vi "view.vi"() -> ()   [LabVIEW 2018]
uses:
  control/clusterCustomString.ctl
  <vilib>/Utility/miscctls.llb/LVPointTypeDef.ctl
  control/enumFgvFunction.ctl
  control/enumTcpCommand.ctl
  <vilib>/Utility/sysdir.llb/System Directory Type.ctl
  control/clusterPeriod.ctl
panel:
  out "Get Whisper(Recv ms)":u32(graph)
  in  "File Name":string
  in  "Save":bool
  out "connect?":bool
  out "rx(ms)":u32
  out "tx(ms)":u32
  out "retry":i32
  in  "Tab Control":enum32{"monitor1", "monitor2", "RecipeLab"}(tab)
  out "value 1-1":T1[](array[typedef]) {"value" format="%#_6f"}
  out "chart 1-1":dbl[][](graph)
  in  "display 1-1":cluster{"subject":u16}[](array[cluster]) {"subject" items=["current_0", "current_1", "current_2", "current_3", "refSpeed_0", "refSpeed_1", "refSpeed_2", "refSpeed_3", "in_rpm_0", "in_rpm_1", "in_rpm_2", "in_rpm_3", "out_rpm_0", "out_rpm_1", "out_rpm_2", "out_rpm_3", "temperature_0", "temperature_1", "temperature_2", "temperature_3", "position_0", "position_1", "position_2", "position_3", "", "", "", "", "", ""]}
  out "chart 1-2":dbl[][](graph)
  out "value 1-2":T1[](array[typedef]) {"value" format="%#_6f"}
  in  "display 1-2":cluster{"subject":u16}[](array[cluster]) {"subject" items=["current_0", "current_1", "current_2", "current_3", "refSpeed_0", "refSpeed_1", "refSpeed_2", "refSpeed_3", "in_rpm_0", "in_rpm_1", "in_rpm_2", "in_rpm_3", "out_rpm_0", "out_rpm_1", "out_rpm_2", "out_rpm_3", "temperature_0", "temperature_1", "temperature_2", "temperature_3", "position_0", "position_1", "position_2", "position_3", "", "", "", "", "", ""]}
  out "chart 2-1":dbl[][](graph)
  out "value 2-1":T1[](array[typedef]) {"value" format="%#_6f"}
  in  "display 2-1":cluster{"subject":u16}[](array[cluster])
  out "chart 2-2":dbl[][](graph)
  out "value 2-2":T1[](array[typedef]) {"value" format="%#_6f"}
  in  "display 2-2":cluster{"subject":u16}[](array[cluster])
  out "stop":bool
  out "rx_packet ts":timestamp format="%<%H:%M:%S%3u>T"
  out "tx_packet ts":timestamp format="%<%H:%M:%S%3u>T"
  in  "send":bool
  in  "tcp rx close?":bool
  in  "port":u16=10300
  in  "address":string="127.0.0.1"
  out "rx_packet":string
  out "tx_packet":string
  in  "saving?":bool
  in  "tx string":string
  out "Whisper":T1[](array[typedef]) {"value" format="%#_6f"}
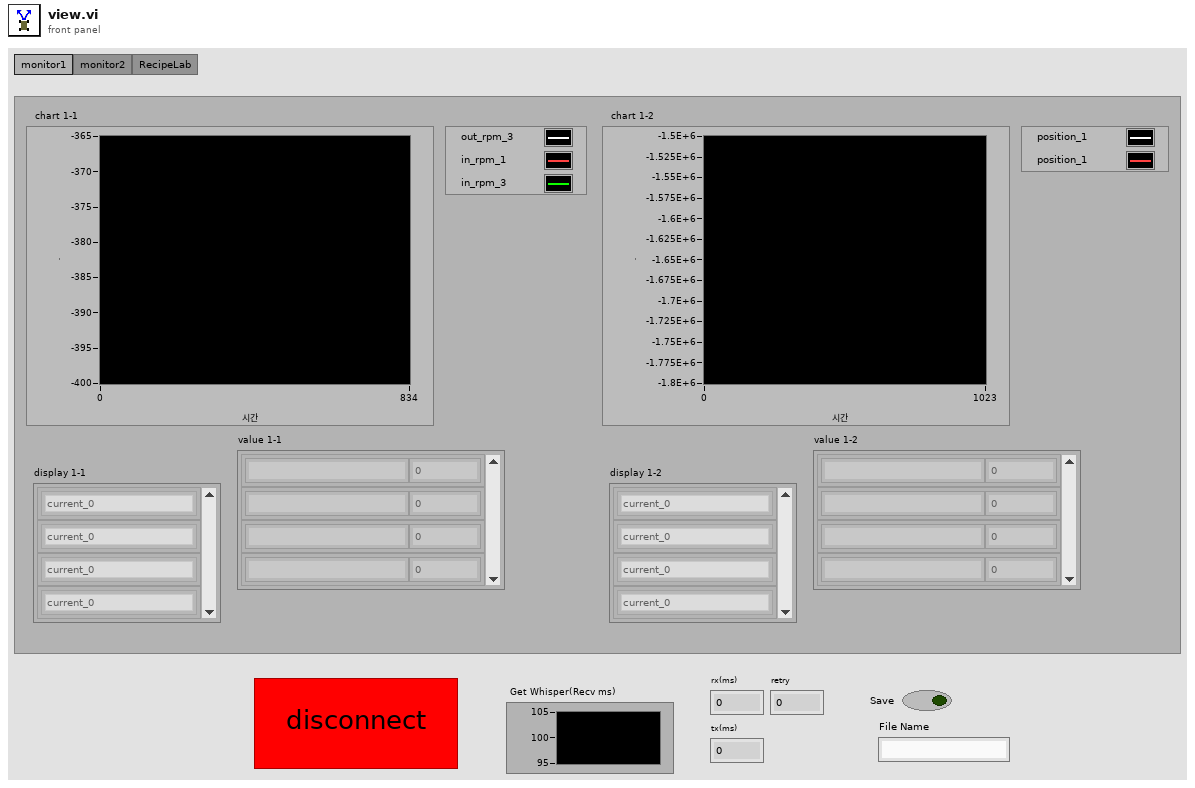
[diagram p1: front panel]
types:
  T1 = typedef "clusterCustomString.ctl" = cluster{"subject":string, "value":dbl}
  T2 = enum32{"invalid app kind", "Development System", "Run Time System", "Student Edition", "Embedded LabVIEW", "Evaluation", "Custom"}
  T3 = typedef "LVPointTypeDef.ctl" = cluster{"Horizontal":i16, "Vertical":i16}
  T4 = typedef "enumFgvFunction.ctl" = enum16{"Open", "Read", "Check", "Write", "Close"}
  T5 = cluster{"subject":u64, "subject":i64, "val_dbl":dbl}[]
  T6 = typedef "System Directory Type.ctl" = i32
  T7 = typedef "clusterPeriod.ctl" = cluster{"Period(ms)":i32}
  T8 = typedef "enumTcpCommand.ctl" = enum16{"None", "Stop", "E-Stop", "Set Position Control Mode", "Set Jog Control Mode", "Set Control Mode", "Set Jog Control Profile Parameter", "Set Position Control Profile Parameter", "Set Jog State", "Set Position", "Start Position Control", "Get Total State", "Get Platform State", "Get Sensor State", "Get Position State", "Init Platform", "Get Whisper State", "Set Sensor"}
  T9 = enum16{"Standard", "Buffered", "CRLF", "Immediate"}
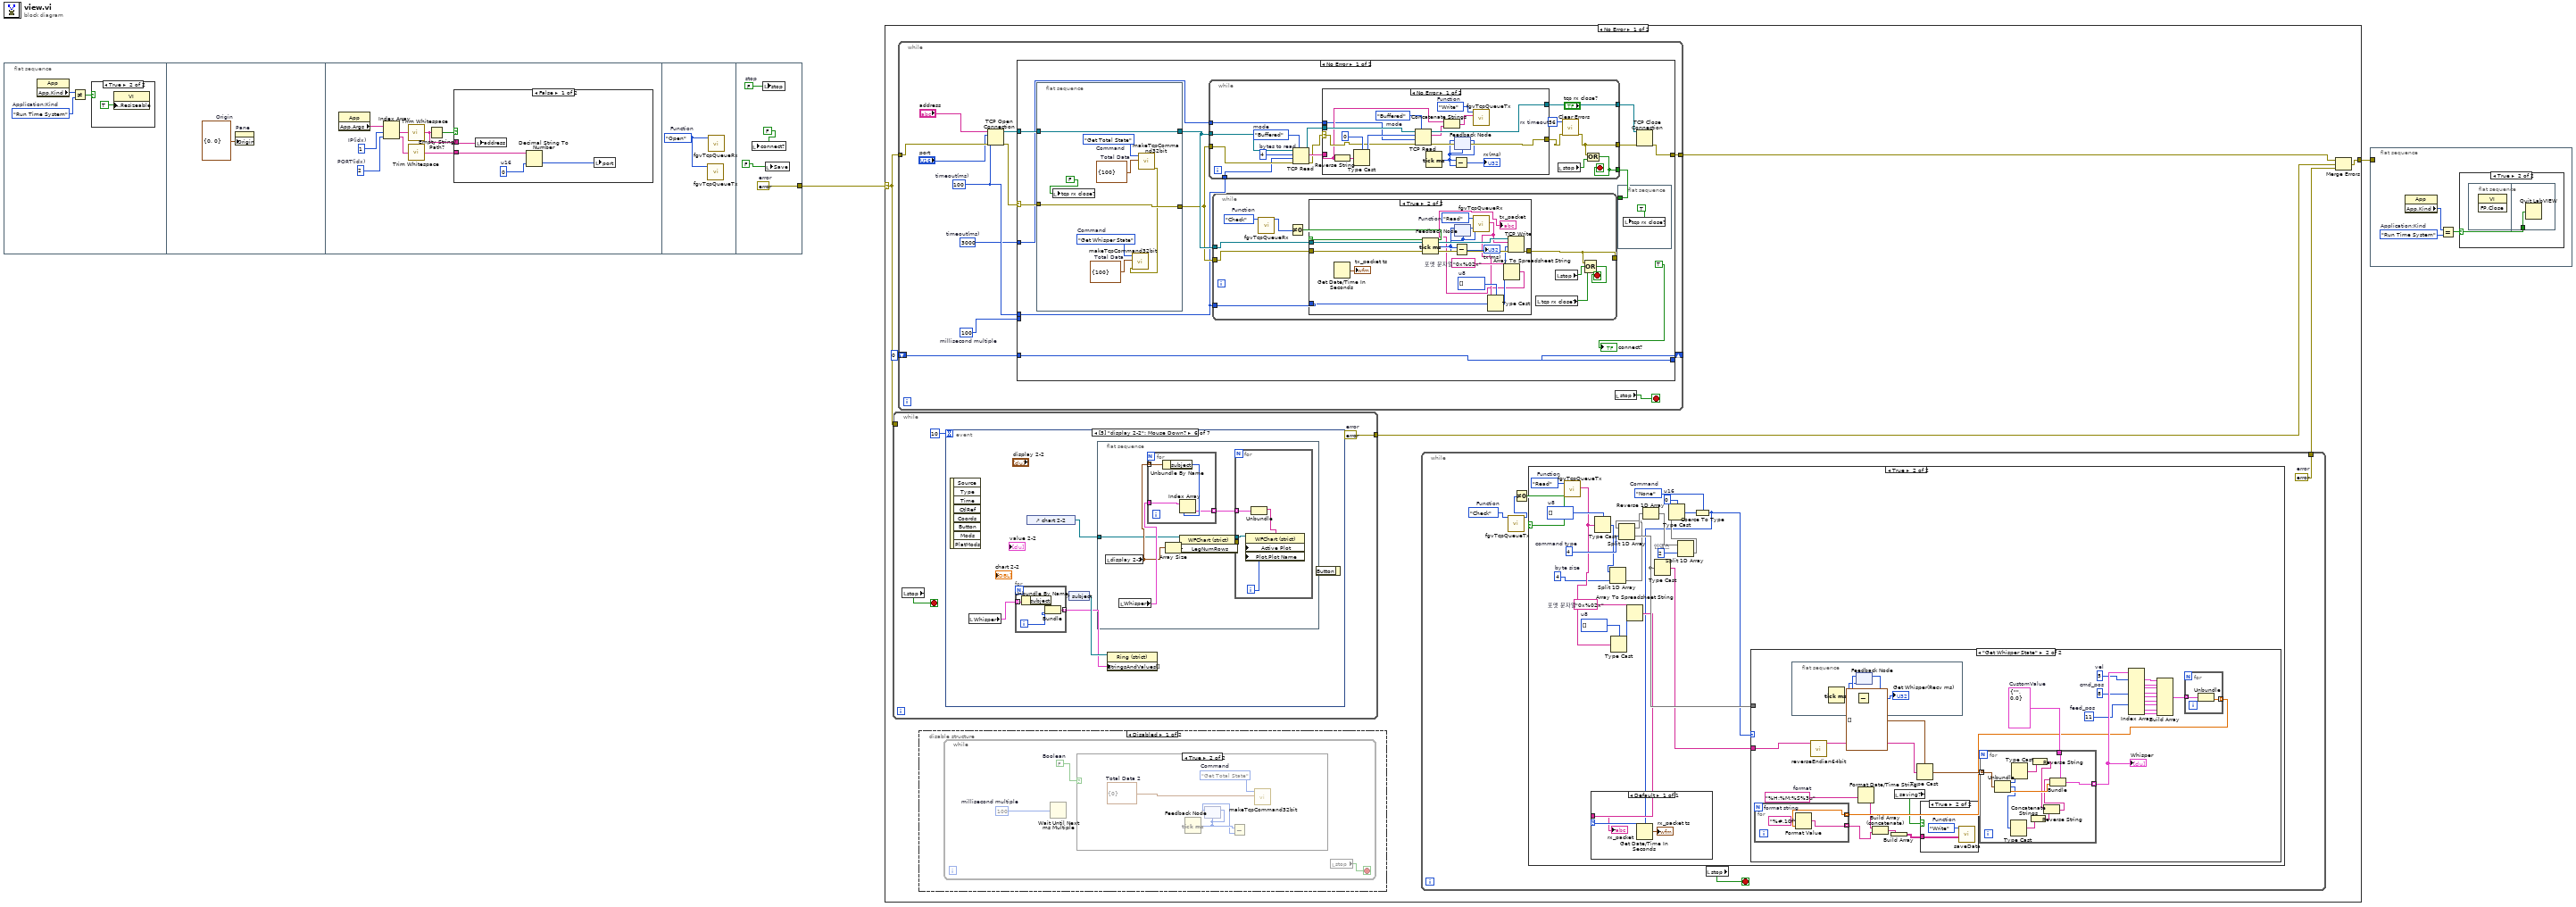
[diagram p0: block diagram]
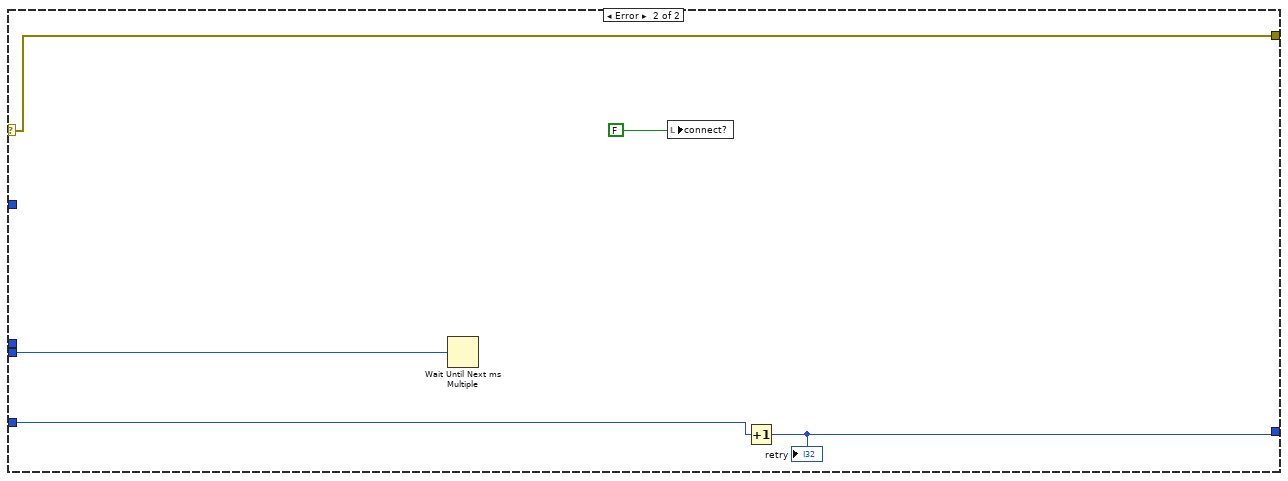
[diagram p9: hidden frame]
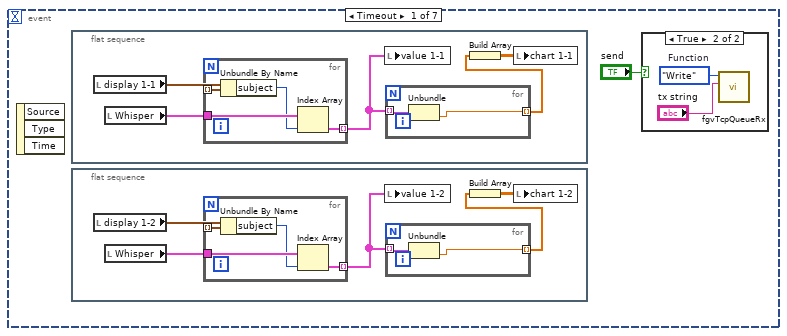
[diagram p10: hidden frame]
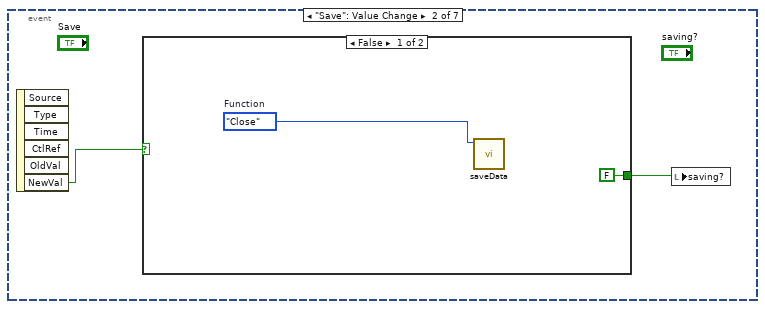
[diagram p12: hidden frame]
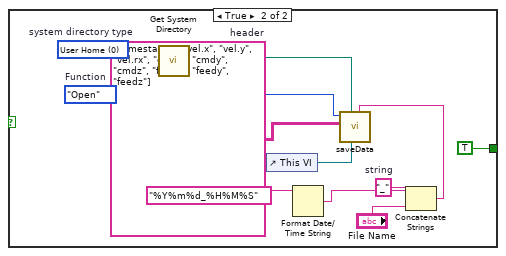
[diagram p13: hidden frame]
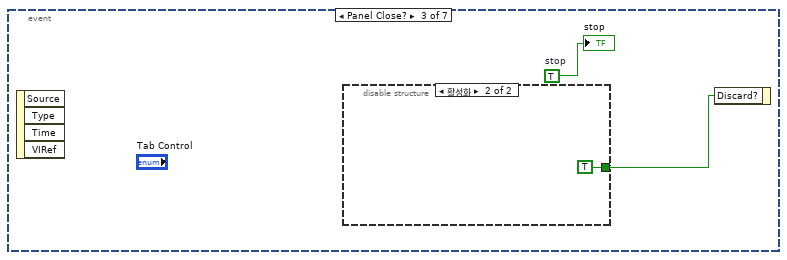
[diagram p14: hidden frame]
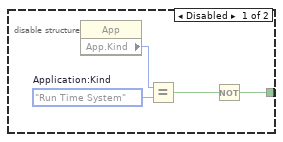
[diagram p15: hidden frame]
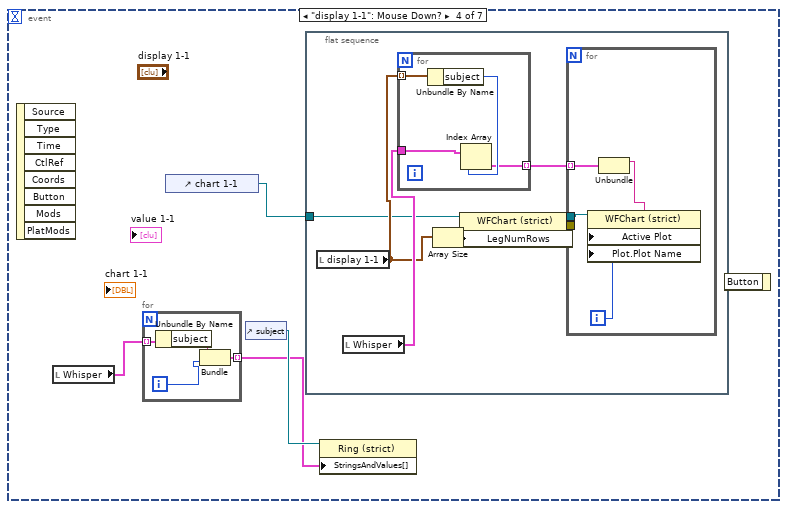
[diagram p16: hidden frame]
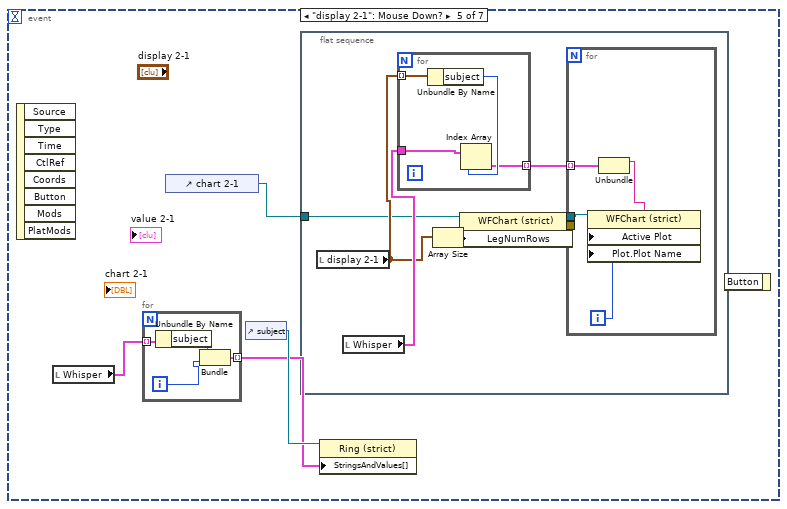
[diagram p17: hidden frame]
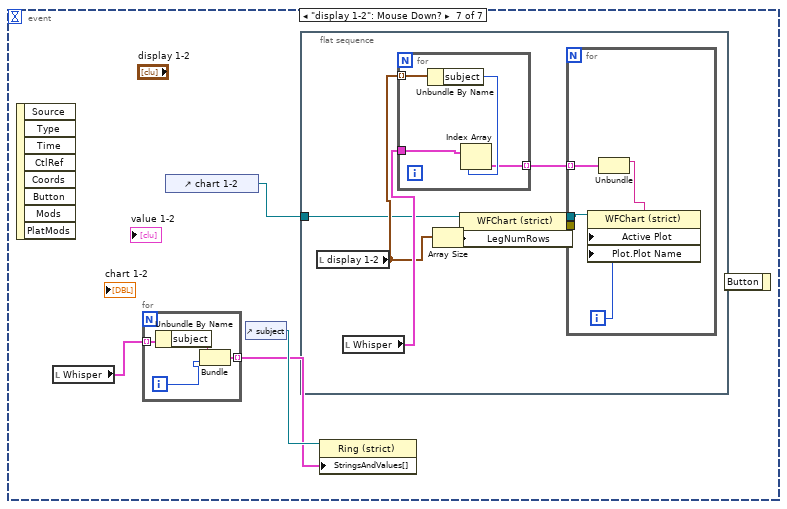
[diagram p18: hidden frame]
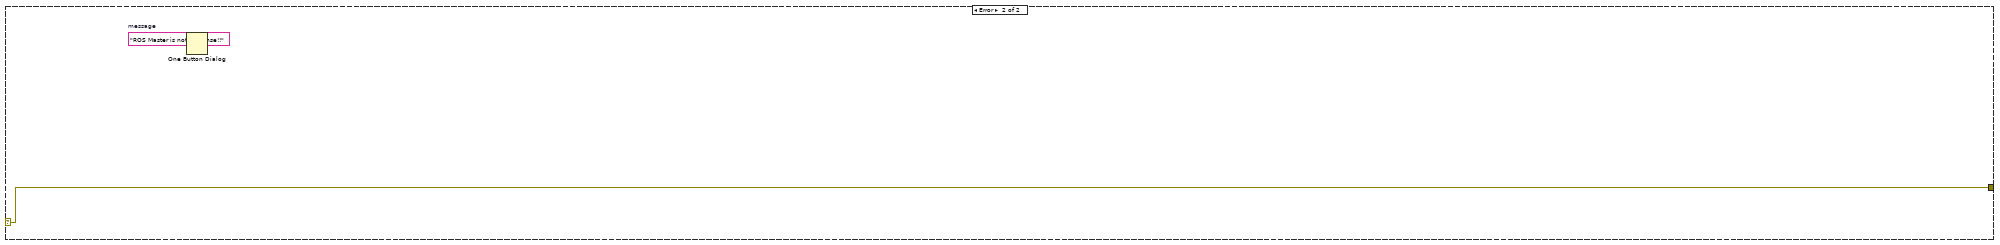
[diagram p19: hidden frame]
diagram:
  n1 = flat-sequence {
    tunnel: [w23] -> w1
    frame #0 {
      w3 = T2."Run Time System"  # Application:Kind
      n2 = property class="App"() -> ("App.Kind"=w4:T2)  [unwired: 2 in, 2 out]
      n3 = Not Equal?(x=w4, y=w3) -> (x != y?=w5:bool)
      n4 = case shown="True" w5 {
        frame False {
        }
        frame True {
          n5 = property class="VI"("Front Panel.Resizeable"=TRUE) -> ()  [unwired: 2 in, 2 out]
        }
      }
    }
    frame #1 {
      w7 = T3 {"Horizontal"=0, "Vertical"=0}  # Origin
      n6 = property on="Pane" class="Pane"("Origin"=w7) -> ()  [unwired: 2 in, 2 out]
    }
    frame #2 {
      w13 = 2  # PORT(idx)
      w14 = 1  # IP(idx)
      n7 = property class="App"() -> ("App.Args"=w15:string[])  [unwired: 2 in, 2 out]
      n8 = Index Array(array=w15, index #1=w14, index #2=w13) -> (element #1=w12:string, element #2=w11:string)
      n9 = call <vilib>:"Trim Whitespace.vi"("string"=w12) -> ("trimmed string"=w10:string)  [unwired: 1 in]
      n10 = call <vilib>:"Trim Whitespace.vi"("string"=w11) -> ("trimmed string"=w9:string)  [unwired: 1 in]
      n11 = Empty String/Path?(string/path=w10) -> (empty?=w8:bool)
      n12 = case shown="False" w8 {
        tunnel: w10 -> [w19 _]
        tunnel: w9 -> [w18 _]
        frame False {
          w16 = u16 0  # u16
          n13 = local write "address"(w19) -> ()
          n14 = Decimal String To Number(string=w18, default (0L)=w16) -> (number=w17:u16)  [unwired: 1 in, 1 out]
          n15 = local write "port"(w17) -> ()
        }
        frame True {
        }
      }
    }
    frame #3 {
      w20 = enumFgvFunction."Open"  # Function
      n16 = call "fgvTcpQueueTx.vi"("Function"=w20) -> ()  [unwired: 8 in, 3 out]
      n17 = call "fgvTcpQueueRx.vi"("Function"=w20) -> ()  [unwired: 8 in, 3 out]
    }
    frame #4 {
      w23 = errorcluster {"status"=FALSE, "code"=0, "source"=""}  # error
      w24 = FALSE  # stop
      n18 = local write "connect?"(FALSE) -> ()
      n19 = local write "stop"(w24) -> ()
      n20 = local write "Save"(FALSE) -> ()
    }
  }
  n21 = case shown="No Error" w1 {
    selector: w1 -> [w28 w348]
    tunnel: [w29 w348] -> w2
    frame No Error {
      n22 = while {
        tunnel: w28 -> [_]
        tunnel: [w209] -> w30
        stop <- w211 stop-if-true
        w209 = errorcluster {"status"=FALSE, "code"=0, "source"=""}  # error
        n23 = local read "stop"() -> (w211:bool)
        n24 = event shown="[5] \"display 2-2\": Mouse Down?" {
          selector: _ -> [_ _ _ _ _ _ _]
          dyn-events: _ -> [_ _ _ _ _ _ _]
          timeout: 10 -> [_ _ _ _ _ _ _]
          event Timeout {
            n25 = event-data() -> ()  [unwired: 1 in, 3 out]
            n26 = flat-sequence {
              frame #0 {
                n27 = local read "display 1-1"() -> (w228:cluster{"subject":u16}[])
                n28 = local read "Whisper"() -> (w227:T1[])
                n29 = for {
                  tunnel: w228 -> [w233] mode=indexing
                  tunnel: w227 -> [w234]
                  tunnel: [w231] -> w225 mode=indexing
                  n30 = Unbundle By Name(w233) -> ("subject"=w232:u16)
                  n31 = Index Array(array=w234, index=w232) -> (element=w231:T1)
                }
                n32 = local write "value 1-1"(w225) -> ()
                n33 = for {
                  tunnel: w225 -> [w230] mode=indexing
                  tunnel: [w229] -> w226 mode=indexing
                  n34 = Unbundle(w230) -> ("value"=w229:dbl)  [unwired: 1 out]
                }
                n35 = Build Array(w226) -> (w224:dbl[][])
                n36 = local write "chart 1-1"(w224) -> ()
              }
            }
            n37 = flat-sequence {
              frame #0 {
                n38 = local read "display 1-2"() -> (w217:cluster{"subject":u16}[])
                n39 = local read "Whisper"() -> (w216:T1[])
                n40 = for {
                  tunnel: w217 -> [w222] mode=indexing
                  tunnel: w216 -> [w223]
                  tunnel: [w220] -> w214 mode=indexing
                  n41 = Unbundle By Name(w222) -> ("subject"=w221:u16)
                  n42 = Index Array(array=w223, index=w221) -> (element=w220:T1)
                }
                n43 = local write "value 1-2"(w214) -> ()
                n44 = for {
                  tunnel: w214 -> [w219] mode=indexing
                  tunnel: [w218] -> w215 mode=indexing
                  n45 = Unbundle(w219) -> ("value"=w218:dbl)  [unwired: 1 out]
                }
                n46 = Build Array(w215) -> (w213:dbl[][])
                n47 = local write "chart 1-2"(w213) -> ()
              }
            }
            n48 = case shown="True" "send" {
              frame False {
              }
              frame True {
                w236 = enumFgvFunction."Write"  # Function
                n49 = call "fgvTcpQueueRx.vi"("Write"="tx string", "Function"=w236) -> ()  [unwired: 7 in, 3 out]
              }
            }
          }
          event "Save": Value Change {
            n50 = event-data() -> ("NewVal"=w238:bool)  [unwired: 1 in, 5 out]
            n51 = case shown="False" w238 {
              tunnel: [FALSE TRUE] -> w237
              frame False {
                w240 = enumFgvFunction."Close"  # Function
                n52 = call "saveData.vi"("Function"=w240) -> ()  [unwired: 8 in, 3 out]
              }
              frame True {
                w241 = "_"  # string
                w246 = string[][] [["timestamp", "vel.x", "vel.y", "vel.rx", "cmdx", "cmdy", "cmdz", "feedx", "feedy", "feedz"]]  # header
                w249 = T6 0 items=["User Home"=0, "User Desktop"=1, "User Documents"=2, "User Application Data"=3, "User Preferences"=4, "User Temporary"=5, "Public Documents"=6, "Public Application Data"=7, "Public Preferences"=8, "Public Cache"=13, "System Core Libraries"=9, "System Installed Libraries"=10, "Application Files"=11, "Boot Volume Root"=12]  # system directory type
                w251 = enumFgvFunction."Open"  # Function
                n53 = call <vilib>:"Get System Directory.vi"("system directory type"=w249) -> ("system directory"=w248:path)  [unwired: 10 in]
                n54 = control-ref of="This VI"() -> (w245:refnum<vi>)
                n55 = Format Date/Time String(time format string (%c)="%Y%m%d_%H%M%S") -> (date/time string=w244:string)  [unwired: 2 in]
                n56 = Concatenate Strings(w244, w241, "File Name") -> (w242:string)
                n57 = call "saveData.vi"("file name"=w242, "이미지 저장 VI"=w245, "file path 경로"=w248, "header"=w246, "Function"=w251) -> ()  [unwired: 4 in, 3 out]
              }
            }
            n58 = local write "saving?"(w237) -> ()
          }
          event Panel Close? {
            w252 = TRUE  # stop
            n59 = event-data() -> ()  [unwired: 1 in, 4 out]
            n60 = disable-structure shown="활성화" {
              disable-tunnel: [w254 TRUE] -> w253
              frame Disabled {
                w256 = T2."Run Time System"  # Application:Kind
                n61 = property class="App"() -> ("App.Kind"=w257:T2)  [unwired: 2 in, 2 out]
                n62 = Equal?(x=w257, y=w256) -> (x = y?=w255:bool)
                n63 = Not(x=w255) -> (.not. x?=w254:bool)
              }
              frame Enabled {
              }
            }
            n64 = event-data("Discard?"=w253) -> ()  [unwired: 1 in, 1 out]
            "stop" <- w252
          }
          event "display 1-1": Mouse Down? {
            n65 = event-data() -> ()  [unwired: 1 in, 8 out]
            n66 = local read "Whisper"() -> (w261:T1[])
            n67 = for {
              tunnel: [w278] -> w260 mode=indexing
              tunnel: w261 -> [w277] mode=indexing
              i -> [w279]
              n68 = Unbundle By Name(w277) -> ("subject"=w280:string)
              n69 = Bundle("subject"=w280, w279) -> (w278:cluster{"subject":string, i32})  [unwired: 1 in]
            }
            n70 = control-ref of="chart 1-1"() -> (w259:refnum<vi>)
            n71 = control-ref of="subject"() -> (w262:refnum<vi>)
            n72 = flat-sequence {
              tunnel: w259 -> [w263]
              frame #0 {
                n73 = local read "display 1-1"() -> (w265:cluster{"subject":u16}[])
                n74 = local read "Whisper"() -> (w266:T1[])
                n75 = for {
                  tunnel: w265 -> [w271] mode=indexing
                  tunnel: w266 -> [w272]
                  tunnel: [w269] -> w264 mode=indexing
                  n76 = Unbundle By Name(w271) -> ("subject"=w270:u16)
                  n77 = Index Array(array=w272, index=w270) -> (element=w269:T1)
                }
                n78 = Array Size(array=w265) -> (size(s)=w268:i32)
                n79 = property on="프로퍼티 노드" class="WFChart (strict)"(reference=w263, "LegNumRows"=w268) -> (error out=w267:errorcluster)  [unwired: 1 in, 1 out]
                n80 = for {
                  tunnel: w267 -> [_]
                  tunnel: w264 -> [w275] mode=indexing
                  tunnel: w263 -> [w273]
                  i -> [w276]
                  n81 = Unbundle(w275) -> ("subject"=w274:string)  [unwired: 1 out]
                  n82 = property on="프로퍼티 노드" class="WFChart (strict)"(reference=w273, "Active Plot"=w276, "Plot.Plot Name"=w274) -> ()  [unwired: 1 in, 2 out]
                }
              }
            }
            n83 = property class="Ring (strict)"(reference=w262, "StringsAndValues[]"=w260) -> ()  [unwired: 1 in, 2 out]
            n84 = event-data() -> ()  [unwired: 2 in, 1 out]
          }
          event "display 2-1": Mouse Down? {
            n85 = event-data() -> ()  [unwired: 1 in, 8 out]
            n86 = local read "Whisper"() -> (w283:T1[])
            n87 = for {
              tunnel: [w300] -> w282 mode=indexing
              tunnel: w283 -> [w299] mode=indexing
              i -> [w301]
              n88 = Unbundle By Name(w299) -> ("subject"=w302:string)
              n89 = Bundle("subject"=w302, w301) -> (w300:cluster{"subject":string, i32})  [unwired: 1 in]
            }
            n90 = control-ref of="chart 2-1"() -> (w281:refnum<vi>)
            n91 = control-ref of="subject"() -> (w284:refnum<vi>)
            n92 = flat-sequence {
              tunnel: w281 -> [w285]
              frame #0 {
                n93 = local read "display 2-1"() -> (w287:cluster{"subject":u16}[])
                n94 = local read "Whisper"() -> (w288:T1[])
                n95 = for {
                  tunnel: w287 -> [w293] mode=indexing
                  tunnel: w288 -> [w294]
                  tunnel: [w291] -> w286 mode=indexing
                  n96 = Unbundle By Name(w293) -> ("subject"=w292:u16)
                  n97 = Index Array(array=w294, index=w292) -> (element=w291:T1)
                }
                n98 = Array Size(array=w287) -> (size(s)=w290:i32)
                n99 = property on="프로퍼티 노드" class="WFChart (strict)"(reference=w285, "LegNumRows"=w290) -> (error out=w289:errorcluster)  [unwired: 1 in, 1 out]
                n100 = for {
                  tunnel: w289 -> [_]
                  tunnel: w286 -> [w297] mode=indexing
                  tunnel: w285 -> [w295]
                  i -> [w298]
                  n101 = Unbundle(w297) -> ("subject"=w296:string)  [unwired: 1 out]
                  n102 = property on="프로퍼티 노드" class="WFChart (strict)"(reference=w295, "Active Plot"=w298, "Plot.Plot Name"=w296) -> ()  [unwired: 1 in, 2 out]
                }
              }
            }
            n103 = property class="Ring (strict)"(reference=w284, "StringsAndValues[]"=w282) -> ()  [unwired: 1 in, 2 out]
            n104 = event-data() -> ()  [unwired: 2 in, 1 out]
          }
          event "display 2-2": Mouse Down? {
            n105 = event-data() -> ()  [unwired: 1 in, 8 out]
            n106 = local read "Whisper"() -> (w305:T1[])
            n107 = for {
              tunnel: [w322] -> w304 mode=indexing
              tunnel: w305 -> [w321] mode=indexing
              i -> [w323]
              n108 = Unbundle By Name(w321) -> ("subject"=w324:string)
              n109 = Bundle("subject"=w324, w323) -> (w322:cluster{"subject":string, i32})  [unwired: 1 in]
            }
            n110 = control-ref of="chart 2-2"() -> (w303:refnum<vi>)
            n111 = control-ref of="subject"() -> (w306:refnum<vi>)
            n112 = flat-sequence {
              tunnel: w303 -> [w307]
              frame #0 {
                n113 = local read "display 2-2"() -> (w309:cluster{"subject":u16}[])
                n114 = local read "Whisper"() -> (w310:T1[])
                n115 = for {
                  tunnel: w309 -> [w315] mode=indexing
                  tunnel: w310 -> [w316]
                  tunnel: [w313] -> w308 mode=indexing
                  n116 = Unbundle By Name(w315) -> ("subject"=w314:u16)
                  n117 = Index Array(array=w316, index=w314) -> (element=w313:T1)
                }
                n118 = Array Size(array=w309) -> (size(s)=w312:i32)
                n119 = property on="프로퍼티 노드" class="WFChart (strict)"(reference=w307, "LegNumRows"=w312) -> (error out=w311:errorcluster)  [unwired: 1 in, 1 out]
                n120 = for {
                  tunnel: w311 -> [_]
                  tunnel: w308 -> [w319] mode=indexing
                  tunnel: w307 -> [w317]
                  i -> [w320]
                  n121 = Unbundle(w319) -> ("subject"=w318:string)  [unwired: 1 out]
                  n122 = property on="프로퍼티 노드" class="WFChart (strict)"(reference=w317, "Active Plot"=w320, "Plot.Plot Name"=w318) -> ()  [unwired: 1 in, 2 out]
                }
              }
            }
            n123 = property class="Ring (strict)"(reference=w306, "StringsAndValues[]"=w304) -> ()  [unwired: 1 in, 2 out]
            n124 = event-data() -> ()  [unwired: 2 in, 1 out]
          }
          event "display 1-2": Mouse Down? {
            n125 = event-data() -> ()  [unwired: 1 in, 8 out]
            n126 = local read "Whisper"() -> (w327:T1[])
            n127 = for {
              tunnel: [w344] -> w326 mode=indexing
              tunnel: w327 -> [w343] mode=indexing
              i -> [w345]
              n128 = Unbundle By Name(w343) -> ("subject"=w346:string)
              n129 = Bundle("subject"=w346, w345) -> (w344:cluster{"subject":string, i32})  [unwired: 1 in]
            }
            n130 = control-ref of="chart 1-2"() -> (w325:refnum<vi>)
            n131 = control-ref of="subject"() -> (w328:refnum<vi>)
            n132 = flat-sequence {
              tunnel: w325 -> [w329]
              frame #0 {
                n133 = local read "display 1-2"() -> (w331:cluster{"subject":u16}[])
                n134 = local read "Whisper"() -> (w332:T1[])
                n135 = for {
                  tunnel: w331 -> [w337] mode=indexing
                  tunnel: w332 -> [w338]
                  tunnel: [w335] -> w330 mode=indexing
                  n136 = Unbundle By Name(w337) -> ("subject"=w336:u16)
                  n137 = Index Array(array=w338, index=w336) -> (element=w335:T1)
                }
                n138 = Array Size(array=w331) -> (size(s)=w334:i32)
                n139 = property on="프로퍼티 노드" class="WFChart (strict)"(reference=w329, "LegNumRows"=w334) -> (error out=w333:errorcluster)  [unwired: 1 in, 1 out]
                n140 = for {
                  tunnel: w333 -> [_]
                  tunnel: w330 -> [w341] mode=indexing
                  tunnel: w329 -> [w339]
                  i -> [w342]
                  n141 = Unbundle(w341) -> ("subject"=w340:string)  [unwired: 1 out]
                  n142 = property on="프로퍼티 노드" class="WFChart (strict)"(reference=w339, "Active Plot"=w342, "Plot.Plot Name"=w340) -> ()  [unwired: 1 in, 2 out]
                }
              }
            }
            n143 = property class="Ring (strict)"(reference=w328, "StringsAndValues[]"=w326) -> ()  [unwired: 1 in, 2 out]
            n144 = event-data() -> ()  [unwired: 2 in, 1 out]
          }
        }
      }
      n145 = while {
        tunnel: w28 -> [w123]
        tunnel: [w122] -> w27
        shift-right: [w117] -> _
        shift-left: 0 -> [w116]
        stop <- w124 stop-if-true
        w113 = 3000  # timeout(ms)
        w115 = u32 100  # millisecond multiple
        w114 = 100  # timeout(ms)
        n146 = TCP Open Connection(address="address", remote port or service name="port", timeout ms (60000)=w114, error in (no error)=w123) -> (connection ID=w119:refnum<k5>, error out=w118:errorcluster)  [unwired: 1 in]
        n147 = case shown="No Error" w118 {
          selector: w118 -> [w128 w208]
          tunnel: [w135 w208] -> w122
          tunnel: w119 -> [w130 _]
          tunnel: [w133 w206] -> w117
          tunnel: w116 -> [w133 w207]
          tunnel: w115 -> [_ w204]
          tunnel: w114 -> [w127 _]
          tunnel: w113 -> [w126 _]
          frame No Error {
            n148 = flat-sequence {
              tunnel: [w145] -> w131
              tunnel: w130 -> [w145]
              tunnel: [w144] -> w129
              tunnel: w128 -> [w144]
              frame #0 {
                w141 = T7 {"Period(ms)"=100}  # Total Data
                w140 = enumTcpCommand."Get Whisper State"  # Command
                w142 = T7 {"Period(ms)"=100}  # Total Data
                w143 = enumTcpCommand."Get Total State"  # Command
                n149 = local write "tcp rx close?"(FALSE) -> ()
                n150 = call "makeTcpCommand32bit.vi"("Variant"=w142, "Command"=w143) -> ("error out"=w139:errorcluster)  [unwired: 7 in, 2 out]
                n151 = call "makeTcpCommand32bit.vi"("error in"=w139, "Variant"=w141, "Command"=w140) -> ()  [unwired: 6 in, 3 out]
              }
            }
            n152 = while {
              tunnel: w129 -> [w185]
              tunnel: [w175] -> w136
              tunnel: w131 -> [w184]
              tunnel: [w178] -> w134
              tunnel: w127 -> [w173]
              tunnel: w126 -> [w172]
              tunnel: [w171] -> w125
              stop <- w171 stop-if-true
              w174 = 56  # rx timeout
              w182 = 4  # bytes to read
              w183 = T9."Buffered"  # mode
              n153 = TCP Read(connection ID=w184, bytes to read=w182, error in (no error)=w185, 7:w183, 9:w173) -> (connection ID out=w180:refnum<k5>, data out=w179:string, error out=w177:errorcluster)
              n154 = case shown="No Error" w177 {
                selector: w177 -> [w193 w203]
                tunnel: w180 -> [w200 w202]
                tunnel: w179 -> [w189 _]
                tunnel: [w196 w202] -> w178
                tunnel: [w195 w203] -> w176
                tunnel: w172 -> [w186 _]
                frame No Error {
                  w194 = enumFgvFunction."Write"  # Function
                  w201 = T9."Buffered"  # mode
                  n155 = Reverse String(1:w189) -> (0:w199:string)
                  n156 = Type Cast(type=0, x=w199) -> (*(type *) &x=w198:i32)
                  n157 = TCP Read(connection ID=w200, bytes to read=w198, error in (no error)=w193, 7:w201, 9:w186) -> (connection ID out=w196:refnum<k5>, data out=w188:string, error out=w195:errorcluster)
                  n158 = Tick Count (ms)() -> (millisecond timer value=w191:u32)
                  n159 = Concatenate Strings(w189, w188) -> (w187:string)
                  n160 = feedback #1(w191) -> (w190:u32)
                  n161 = Subtract(x=w191, y=w190) -> (x-y=→"rx(ms)":u32)
                  n162 = feedback-in #1(w191) -> ()
                  n163 = call "fgvTcpQueueTx.vi"("Write"=w187, "Function"=w194) -> ()  [unwired: 7 in, 3 out]
                }
                frame Error {
                }
              }
              n164 = local read "stop"() -> (w181:bool)
              n165 = call <vilib>:"Clear Errors.vi"("error in (no error)"=w176, "specific error code to clear (0: all)"=w174) -> ("error out"=w175:errorcluster)  [unwired: 4 in, 1 out]
              n166 = Compound Arithmetic op=OR(w175, w181) -> (w171:bool)
            }
            n167 = while {
              tunnel: w129 -> [w147]
              tunnel: [w155] -> _
              tunnel: w131 -> [w149]
              tunnel: w127 -> [w148]
              stop <- w153 stop-if-true
              w152 = enumFgvFunction."Check"  # Function
              n168 = call "fgvTcpQueueRx.vi"("Function"=w152) -> ("Count"=w151:i32)  [unwired: 8 in, 2 out]
              n169 = Not Equal To 0?(x=w151) -> (x != 0?=w150:bool)
              n170 = case shown="True" w150 {
                tunnel: [w156 w170] -> w155
                tunnel: w147 -> [w156 w169]
                tunnel: w149 -> [_ w168]
                tunnel: w148 -> [_ w158]
                frame False {
                }
                frame True {
                  w163 = "0x%02x"  # 포맷 문자열
                  w161 = u8[] []  # u8
                  w167 = enumFgvFunction."Read"  # Function
                  n171 = Get Date/Time In Seconds() -> (seconds since 1Jan1904=→"tx_packet ts":timestamp)
                  n172 = Tick Count (ms)() -> (millisecond timer value=w165:u32)
                  n173 = feedback #2(w165) -> (w164:u32)
                  n174 = Subtract(x=w165, y=w164) -> (x-y=→"tx(ms)":u32)
                  n175 = feedback-in #2(w165) -> ()
                  n176 = call "fgvTcpQueueRx.vi"("Function"=w167) -> ("Read"=w160:string)  [unwired: 8 in, 2 out]
                  n177 = Type Cast(type=w161, x=w160) -> (*(type *) &x=w162:u8[])
                  n178 = Array To Spreadsheet String(array=w162, 3:w163) -> (spreadsheet string=→"tx_packet":string)  [unwired: 1 in]
                  n179 = TCP Write(connection ID=w168, data in=w160, error in (no error)=w169, 9:w158) -> (error out=w170:errorcluster)  [unwired: 2 out]
                }
              }
              n180 = local read "tcp rx close?"() -> (w146:bool)
              n181 = local read "stop"() -> (w154:bool)
              n182 = Compound Arithmetic op=OR(w155, w154, w146) -> (w153:bool)
            }
            n183 = flat-sequence {
              tunnel: w125 -> [_]
              frame #0 {
                n184 = local write "tcp rx close?"(TRUE) -> ()
              }
            }
            n185 = TCP Close Connection(connection ID=w134, error in (no error)=w136) -> (error out=w135:errorcluster)  [unwired: 1 in, 1 out]
            "connect?" <- TRUE
          }
          frame Error {
            n186 = Wait Until Next ms Multiple(millisecond multiple=w204) -> ()  [unwired: 1 out]
            n187 = local write "connect?"(FALSE) -> ()
            n188 = Increment(x=w207) -> (x+1=w206:i32)
            "retry" <- w206
          }
        }
        n189 = local read "stop"() -> (w124:bool)
      }
      n190 = disable-structure shown="Disabled" {
        frame Disabled {
          n191 = while {
            stop <- w32 stop-if-true
            w31 = FALSE  # Boolean
            w33 = u32 100  # millisecond multiple
            n192 = Wait Until Next ms Multiple(millisecond multiple=w33) -> ()  [unwired: 1 out]
            n193 = case shown="True" w31 {
              frame False {
              }
              frame True {
                w37 = T7 {"Period(ms)"=0}  # Total Data 2
                w36 = enumTcpCommand."Get Total State"  # Command
                n194 = Tick Count (ms)() -> (millisecond timer value=w35:u32)
                n195 = feedback-in #3(w35) -> ()
                n196 = feedback #3(w35) -> (w34:u32)
                n197 = Subtract(x=w35, y=w34) -> ()  [unwired: 1 out]
                n198 = call "makeTcpCommand32bit.vi"("Variant"=w37, "Command"=w36) -> ()  [unwired: 7 in, 3 out]
              }
            }
            n199 = local read "stop"() -> (w32:bool)
          }
        }
        frame Enabled {
        }
      }
      n200 = while {
        tunnel: [w38] -> w25
        stop <- w41 stop-if-true
        w38 = errorcluster {"status"=FALSE, "code"=0, "source"=""}  # error
        w42 = enumFgvFunction."Check"  # Function
        n201 = call "fgvTcpQueueTx.vi"("Function"=w42) -> ("Count"=w40:i32)  [unwired: 8 in, 2 out]
        n202 = Not Equal To 0?(x=w40) -> (x != 0?=w39:bool)
        n203 = case shown="True" w39 {
          frame False {
          }
          frame True {
            w46 = 2  # 인덱스
            w48 = 4  # byte size
            w53 = "0x%02x"  # 포맷 문자열
            w55 = u8[] []  # u8
            w44 = u16 0  # u16
            w59 = enumTcpCommand."None"  # Command
            w61 = 4  # command type
            w62 = u8[] []  # u8
            w63 = enumFgvFunction."Read"  # Function
            n204 = call "fgvTcpQueueTx.vi"("Function"=w63) -> ("Read"=w51:string)  [unwired: 8 in, 2 out]
            n205 = Type Cast(type=w62, x=w51) -> (*(type *) &x=w50:u8[])
            n206 = Split 1D Array(array=w50, index=w48) -> (second subarray=w49:u8[])  [unwired: 1 out]
            n207 = Type Cast(type=w55, x=w51) -> (*(type *) &x=w54:u8[])
            n208 = Split 1D Array(array=w49, index=w61) -> (first subarray=w60:u8[], second subarray=w57:u8[])
            n209 = Array To Spreadsheet String(array=w54, 3:w53) -> (spreadsheet string=w52:string)  [unwired: 1 in]
            n210 = Reverse 1D Array(array=w60) -> (reversed array=w47:u8[])
            n211 = Type Cast(x=w57) -> (*(type *) &x=w56:string)  [unwired: 1 in]
            n212 = Split 1D Array(array=w47, index=w46) -> (second subarray=w45:u8[])  [unwired: 1 out]
            n213 = Type Cast(type=w44, x=w45) -> (*(type *) &x=w58:u16)
            n214 = Coerce To Type(0:w58, 1:w59) -> (2:w43:T8)
            n215 = case shown="Default" w43 {
              tunnel: w52 -> [w65]
              frame Default {
                n216 = Get Date/Time In Seconds() -> (seconds since 1Jan1904=→"rx_packet ts":timestamp)
                "rx_packet" <- w65
              }
            }
            n217 = case shown="\"Get Whisper State\"" w43 {
              tunnel: w57 -> [_ _]
              tunnel: w56 -> [_ w91]
              frame Default {
              }
              frame "Get Whisper State" {
                w71 = "%H:%M:%S%3u"  # format
                w83 = 11  # feed_pos
                w84 = 8  # cmd_pos
                w85 = 5  # vel
                w87 = T1 {"subject"="", "value"=0.0}  # CustomValue
                n218 = flat-sequence {
                  frame #0 {
                    n219 = Tick Count (ms)() -> (millisecond timer value=w100:u32)
                    n220 = feedback #4(w100) -> (w101:u32)
                    n221 = Subtract(x=w100, y=w101) -> (x-y=→"Get Whisper(Recv ms)":u32)
                    n222 = feedback-in #4(w100) -> ()
                  }
                }
                n223 = call "reverseEndian64bit.vi"("In"=w91) -> ("Out"=w89:string)  [unwired: 9 in, 1 out]
                n224 = Format Date/Time String(time format string (%c)=w71) -> (date/time string=w70:string)  [unwired: 2 in]
                n225 = local read "saving?"() -> (w66:bool)
                n226 = Type Cast(type=T5 [], x=w89) -> (*(type *) &x=w88:T5)
                n227 = for {
                  tunnel: w88 -> [w112] mode=indexing
                  tunnel: w87 -> [w111]
                  tunnel: [w110] -> w86 mode=indexing
                  n228 = Unbundle(w112) -> ("subject"=w109:u64, "subject"=w103:i64, "val_dbl"=w107:dbl)
                  n229 = Type Cast(x=w103) -> (*(type *) &x=w105:string)  [unwired: 1 in]
                  n230 = Type Cast(x=w109) -> (*(type *) &x=w108:string)  [unwired: 1 in]
                  n231 = Reverse String(1:w105) -> (0:w104:string)
                  n232 = Reverse String(1:w108) -> (0:w106:string)
                  n233 = Concatenate Strings(w106, w104) -> (w102:string)
                  n234 = Bundle(cluster=w111, "subject"=w102, "value"=w107) -> (w110:T1)
                }
                "Whisper" <- w86
                n235 = Index Array(array=w86, index #1=w85, index #4=w84, index #7=w83) -> (element #1=w82:T1, element #2=w81:T1, element #3=w80:T1, element #4=w79:T1, element #5=w78:T1, element #6=w77:T1, element #7=w76:T1, element #8=w75:T1, element #9=w74:T1)  [unwired: 6 in]
                n236 = Build Array(w82, w81, w80, w79, w78, w77, w76, w75, w74) -> (w73:T1[])
                n237 = for {
                  tunnel: w73 -> [w98] mode=indexing
                  tunnel: [w97] -> w72 mode=indexing
                  n238 = Unbundle(w98) -> ("value"=w97:dbl)  [unwired: 1 out]
                }
                n239 = for {
                  tunnel: w72 -> [w96] mode=indexing
                  tunnel: [w94] -> w69 mode=indexing
                  w95 = "%#.10f"  # format string
                  n240 = Format Value(format string=w95, value (0)=w96) -> (output string=w94:string)  [unwired: 1 in]
                }
                n241 = Build Array (concatenate)(w70, w69) -> (w68:string[])
                n242 = Build Array(w68) -> (w67:string[][])
                n243 = case shown="True" w66 {
                  tunnel: w67 -> [_ w92]
                  frame False {
                  }
                  frame True {
                    w93 = enumFgvFunction."Write"  # Function
                    n244 = call "saveData.vi"("body"=w92, "Function"=w93) -> ()  [unwired: 7 in, 3 out]
                  }
                }
              }
            }
          }
        }
        n245 = local read "stop"() -> (w41:bool)
      }
      n246 = Merge Errors(w27, w30, w25) -> (w29:errorcluster)
    }
    frame Error {
      w347 = "ROS Master is not response!!"  # message
      n247 = One Button Dialog(message=w347) -> ()  [unwired: 1 in, 1 out]
    }
  }
  n248 = flat-sequence {
    tunnel: w2 -> [_]
    frame #0 {
      w350 = T2."Run Time System"  # Application:Kind
      n249 = property class="App"() -> ("App.Kind"=w351:T2)  [unwired: 2 in, 2 out]
      n250 = Equal?(x=w351, y=w350) -> (x = y?=w349:bool)
      n251 = case shown="True" w349 {
        selector: w349 -> [_ w352]
        frame False {
        }
        frame True {
          n252 = flat-sequence {
            tunnel: w352 -> [w353]
            frame #0 {
              n253 = invoke class="VI" method="FP.Close"() -> ()  [unwired: 3 in, 3 out]
            }
            frame #1 {
              n254 = Quit LabVIEW(quit? (T)=w353) -> ()
            }
          }
        }
      }
    }
  }
